vi "Read Driver State.vi"(8 "error in (no error)":errorcluster, 11 "Driver in":refnum<class "Driver.lvclass">) -> (0 "error out":errorcluster, 2 "Driver State":T1 {"Slide Right Joystick" min=-1.0 max=1.0 scale=-1.0..1.0; "Rotate Right Joystick" min=-1.0 max=1.0 scale=-1.0..1.0; "Forward Joystick" min=-1.0 max=1.0 scale=-1.0..1.0}, 3 "Driver out":refnum<class "Driver.lvclass">)   [LabVIEW 2014, in "Driver.lvlib" / "Driver.lvclass"]
uses:
  Driver.lvclass
  Driver State.ctl
  Joystick/Joystick Class/Button State.ctl
  Joystick/Joystick Class/Axis State.ctl
  Driver.lvclass/Driver.ctl
  Joystick/Joystick Class/Joystick.lvclass
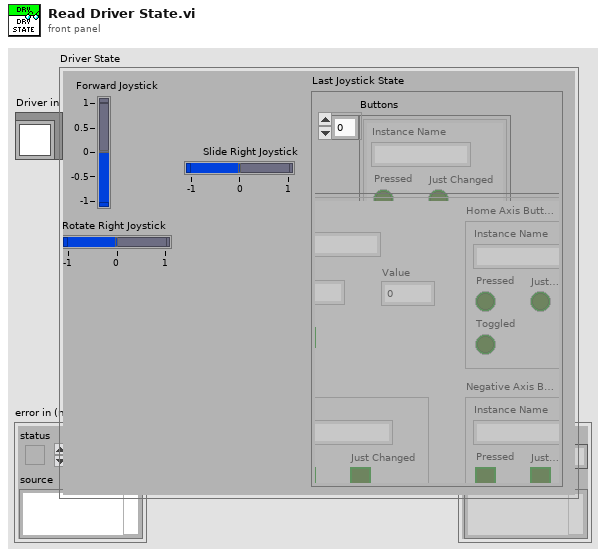
[diagram p1: front panel]
types:
  T1 = typedef "Driver.lvlib/Driver.lvclass/Driver State.ctl" = cluster{"Forward Joystick":dbl, "Rotate Right Joystick":dbl, "Slide Right Joystick":dbl, "Last Joystick State":cluster{"Buttons":T2[], "Axis":T3[]}}
  T2 = typedef "Joystick.lvlib/Joystick.lvclass/Button State.ctl" = cluster{"Pressed":bool, "Instance Name":string, "Toggled":bool, "Just Changed":bool}
  T3 = typedef "Joystick.lvlib/Joystick.lvclass/Axis State.ctl" = cluster{"Instance Name":string, "Deadband":dbl, "Value":dbl, "At Home":bool, "Postive Axis Button State":T2, "Negative Axis Button State":T2, "Home Axis Button State":T2}
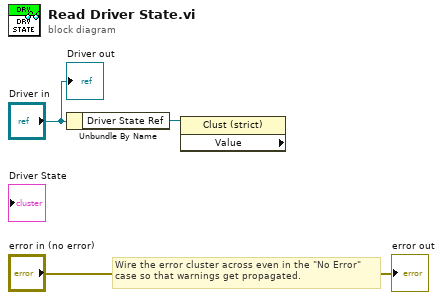
[diagram p0: block diagram]
diagram:
  # "Wire the error cluster across even in the \"No Error\"\ncase so that warnings get propagated."
  n1 = Unbundle By Name("Driver in") -> ("Driver State Ref"=w1:refnum<vi>)
  n2 = property class="Clust (strict)" props=["Value"](reference=w1) -> ()  [unwired: 1 in, 3 out]
  "error out" <- "error in (no error)"
  "Driver out" <- "Driver in"
